vi "InitHardware.vi"(8 "error in (no error)":errorcluster, 11 "NewportXPS in":refnum<class "NewportXPS.lvclass">) -> (0 "error out":errorcluster, 3 "NewportXPS out":refnum<class "NewportXPS.lvclass">)   [LabVIEW 2020, in "NewportXPS.lvclass"]
uses:
  NewportXPS.lvclass
  NewportXPS.lvclass/NewportXPS.ctl
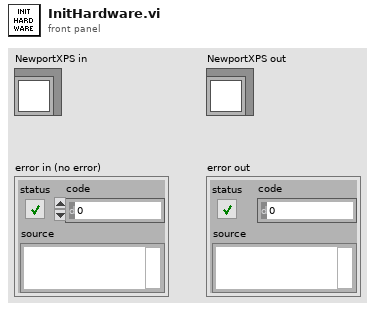
[diagram p1: front panel]
types:
  T1 = cluster{"connection TCP":refnum<k5>, "LogTo File":bool, "Log File refnum":refnum<file>, "no error if error log":bool}
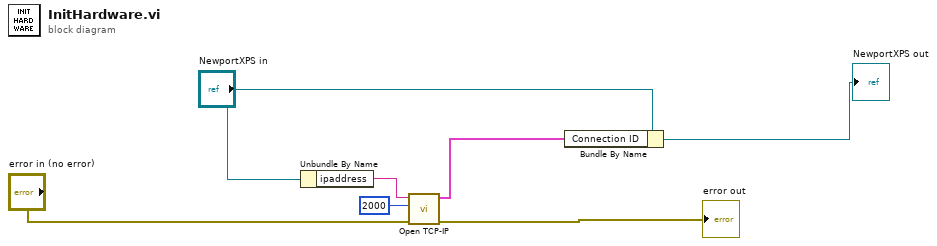
[diagram p0: block diagram]
diagram:
  n1 = Unbundle By Name("NewportXPS in") -> ("ipaddress"=w1:string)
  n2 = call "Open TCP-IP.vi"("error in (no error)"="error in (no error)", "timeout ms (60000)"=2000, "IP address"=w1) -> ("error out"=→"error out":errorcluster, "Connection ID"=w6:T1)  [unwired: 6 in, 1 out]
  n3 = Bundle By Name(cluster="NewportXPS in", "Connection ID"=w6) -> (→"NewportXPS out":refnum<class "NewportXPS.lvclass">)
